vi "Conditional String Concatenate.vi"(7 "Search Start Point":T2, 10 "String Match Details":T1) -> (1 "String Buffer out":string, 2 "Response":string)   [LabVIEW 2017, in "SSH.lvlib"]
doc: "Concatenates the string components differently depending on whether the search is being performed from the start or the end of the response string"
uses:
  SSH.lvlib
  Search Start Point.ctl
  String Match Details.ctl
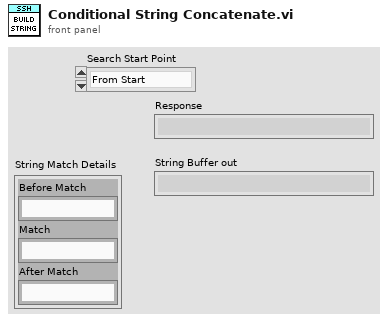
[diagram p1: front panel]
types:
  T1 = typedef "SSH.lvlib/String Match Details.ctl" = cluster{"Before Match":string, "Match":string, "After Match":string}
  T2 = typedef "SSH.lvlib/Search Start Point.ctl" = enum16{"From Start", "From End"}
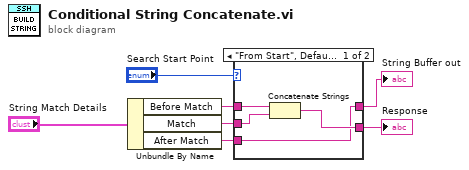
[diagram p0: block diagram]
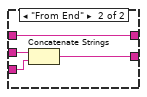
[diagram p2: hidden frame]
diagram:
  n1 = Unbundle By Name("String Match Details") -> ("Before Match"=w3:string, "Match"=w2:string, "After Match"=w1:string)
  n2 = case shown="\"From Start\", Default" "Search Start Point" {
    tunnel: w1 -> [w8 w15]
    tunnel: w2 -> [w10 w14]
    tunnel: [w8 w12] -> w5
    tunnel: w3 -> [w11 w12]
    tunnel: [w9 w13] -> w7
    frame "From Start", Default {
      n3 = Concatenate Strings(w11, w10) -> (w9:string)
    }
    frame "From End" {
      n4 = Concatenate Strings(w14, w15) -> (w13:string)
    }
  }
  "Response" <- w7
  "String Buffer out" <- w5
